vi "Set AWS Credentials.vi"(8 "error in (no error)":errorcluster, 11 "AWS Credentials in":T1) -> (0 "error out":errorcluster)   [LabVIEW 2015, in "LV Interface for Amazon S3.lvlib"]
doc: "<B>Stores the AWS Credentials</B> (AWS Access Key & AWS Secret Key) in a FG. You need to <B>call this VI only once, prior to any Amazon S3 requests</B>. The <B>credentials will be used during all the requests</B> you make to Amazon S3. To obtain AWS Credentials <B>you must first register with Amazon AWS</B>. Because this operation initializes the FG that stores your credentials, <B>you should place this VI in your Top-level VI</B>, or at a place in your VI hierarchy <B>so that you can ensure the FG will not go out of memory</B> while you are using Amazon S3 toolkit VIs."
uses:
  LV Interface for Amazon S3.lvlib
  Typedefs/AMZ_S3_AWS Credentials.ctl
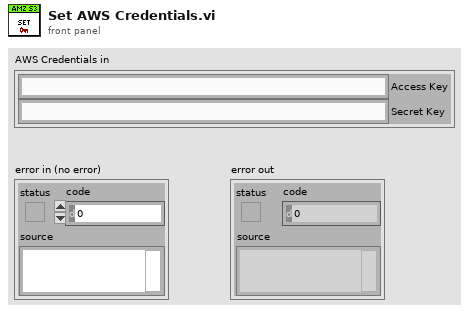
[diagram p1: front panel]
types:
  T1 = typedef "LV Interface for Amazon S3.lvlib/AMZ_S3_AWS Credentials.ctl" = cluster{"Access Key":string, "Secret Key":string}
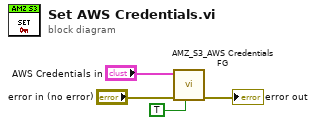
[diagram p0: block diagram]
diagram:
  n1 = call "AMZ_S3_AWS Credentials FG.vi"("Set?"=TRUE, "error in (no error)"="error in (no error)", "AWS Credentials in"="AWS Credentials in") -> ("error out"=→"error out":errorcluster)  [unwired: 7 in, 1 out]
